vi "Nav Waveforms.vi"(10 "Log Data In":cluster{refnum<class "RDS State.lvclass">[]}[](array[cluster]), 11 "Log Header":T1) -> (2 "Log Data Out":cluster{refnum<class "RDS State.lvclass">[]}[](array[cluster]), 3 "Log Header Out":T1, 5 "Nav Data Out":waveform(dbl)[](array[waveform]))   [LabVIEW 2015, in "Log Waveform Processors.lvlib"]
uses:
  Log Waveform Processors.lvlib
  RDS State Tracker/RDS State/RDS State.lvclass
  Actors/RDS Logger Actor/RDS Logger Actor/RDS Logger Actor/Logger Header.ctl
  RDS State Tracker/RDS State/RDS State.lvclass/RDS State.ctl
  <vilib>/measure/maresamp.llb/Resample Waveform (single shot).vi
  <vilib>/Waveform/WDTFileIO.llb/Export Waveforms To Spreadsheet File (1D).vi
  <vilib>/measure/NI_MAPro.lvlib
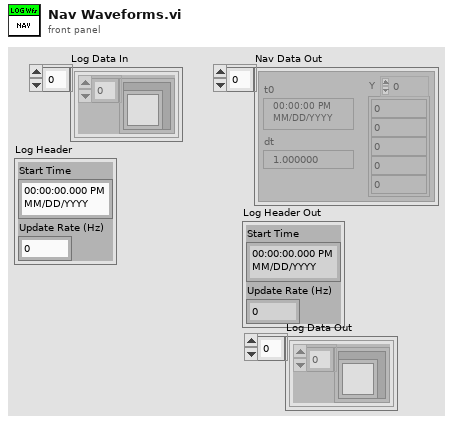
[diagram p1: front panel]
types:
  T1 = typedef "Log Waveform Processors.lvlib/Logger Header.ctl" = cluster{"Start Time":timestamp, "Update Rate (Hz)":dbl}
  T2 = typedef "RDS Libraries.lvlib/NMEA.lvlib/NMEA_GPRMC-data.ctl" = cluster{"TimeStamp":timestamp, "Validity":bool, "Latitude":dbl, "Latitude-Direction":T3, "Longitude":dbl, "Longitude-Direction":T4, "Speed in knots":sgl, "True course":sgl, "Date Stamp":timestamp, "Magnetic Variation (East/West)":sgl, "GPS Latitude":dbl, "GPS Longitude":dbl}
  T3 = typedef "RDS Libraries.lvlib/NMEA.lvlib/NMEA_LatitudeDirection.ctl" = enum16{"", "North", "South"}
  T4 = typedef "RDS Libraries.lvlib/NMEA.lvlib/NMEA_LongitudeDirection.ctl" = enum16{"", "East", "West"}
  T5 = typedef "RDS Instrument Library.lvlib/Compass Data.ctl" = cluster{"Compass Heading":sgl, "pitch Angle":sgl, "roll Angle":sgl, "Temperature":sgl, "Depth":sgl, "Magnetic Field":sgl, "Magnetic Field X":sgl, "Magnetic Field Y":sgl, "Magnetic Field Z":sgl, "Acceleration":sgl, "Acceleration X":sgl, "Acceleration Y":sgl, "Gyro":sgl, "Gyro X":sgl, "Acceleration Z":sgl, "Gyro Y":sgl, "Raw Heading":sgl}
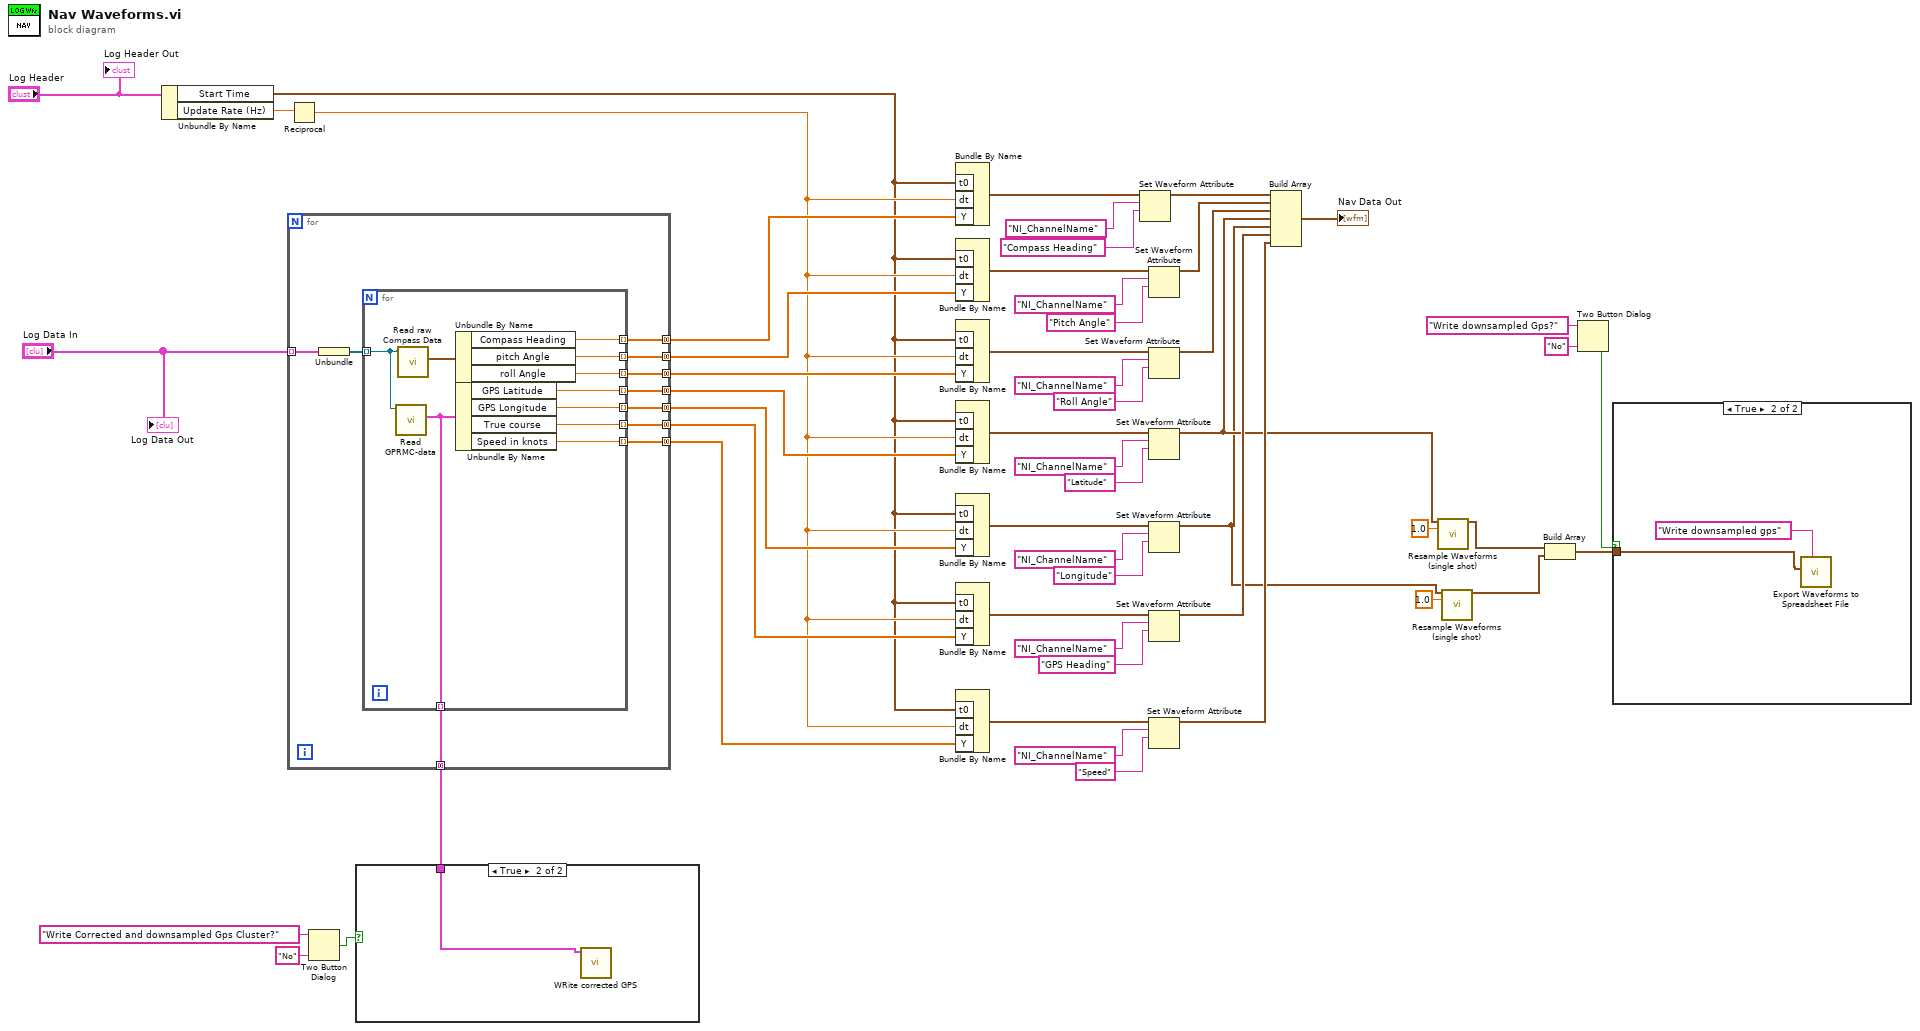
[diagram p0: block diagram]
diagram:
  n1 = Unbundle By Name("Log Header") -> ("Start Time"=w16:timestamp, "Update Rate (Hz)"=w18:dbl)
  n2 = for {
    tunnel: "Log Data In" -> [w63] mode=indexing
    tunnel: [w61] -> w25 mode=concatenating
    tunnel: [w60] -> w30 mode=concatenating
    tunnel: [w59] -> w31 mode=concatenating
    tunnel: [w58] -> w47 mode=concatenating
    tunnel: [w57] -> w48 mode=concatenating
    tunnel: [w56] -> w52 mode=concatenating
    tunnel: [w55] -> w21 mode=concatenating
    tunnel: [w54] -> w7 mode=concatenating
    n3 = Unbundle(w63) -> (w62:refnum<class "RDS State.lvclass">[])
    n4 = for {
      tunnel: w62 -> [w65] mode=indexing
      tunnel: [w73] -> w61 mode=indexing
      tunnel: [w72] -> w60 mode=indexing
      tunnel: [w71] -> w59 mode=indexing
      tunnel: [w69] -> w58 mode=indexing
      tunnel: [w68] -> w57 mode=indexing
      tunnel: [w67] -> w56 mode=indexing
      tunnel: [w66] -> w55 mode=indexing
      tunnel: [w64] -> w54 mode=indexing
      n5 = call "Read GPRMC-data.vi"("RDS State in"=w65) -> ("GPRMC-data"=w64:T2)  [unwired: 8 in, 2 out]
      n6 = call "Read raw Compass Data.vi"("RDS State in"=w65) -> ("Compass Data"=w70:T5)  [unwired: 8 in, 2 out]
      n7 = Unbundle By Name(w70) -> ("Compass Heading"=w73:sgl, "pitch Angle"=w72:sgl, "roll Angle"=w71:sgl)
      n8 = Unbundle By Name(w64) -> ("GPS Latitude"=w69:dbl, "GPS Longitude"=w68:dbl, "True course"=w67:sgl, "Speed in knots"=w66:sgl)
    }
  }
  n9 = Reciprocal(x=w18) -> (1/x=w17:dbl)
  n10 = Two Button Dialog(message="Write Corrected and downsampled Gps Cluster?", 1:"No" ("F button name (\"Cancel\")")) -> (T button?=w6:bool)  [unwired: 1 in]
  n11 = case shown="True" w6 {
    tunnel: w7 -> [_ w74]
    frame False {
    }
    frame True {
      n12 = call "WRite corrected GPS.vi"("Raw GPS Data"=w74) -> ()  [unwired: 11 in]
    }
  }
  n13 = Bundle By Name("t0"=w16, "dt"=w17, "Y"=w25) -> (w26:waveform(sgl))  [unwired: 1 in]
  n14 = Bundle By Name("t0"=w16, "dt"=w17, "Y"=w30) -> (w28:waveform(sgl))  [unwired: 1 in]
  n15 = Bundle By Name("t0"=w16, "dt"=w17, "Y"=w31) -> (w29:waveform(sgl))  [unwired: 1 in]
  n16 = Bundle By Name("t0"=w16, "dt"=w17, "Y"=w47) -> (w43:waveform(dbl))  [unwired: 1 in]
  n17 = Bundle By Name("t0"=w16, "dt"=w17, "Y"=w48) -> (w44:waveform(dbl))  [unwired: 1 in]
  n18 = Bundle By Name("t0"=w16, "dt"=w17, "Y"=w52) -> (w51:waveform(sgl))  [unwired: 1 in]
  n19 = Bundle By Name("t0"=w16, "dt"=w17, "Y"=w21) -> (w22:waveform(sgl))  [unwired: 1 in]
  n20 = Set Waveform Attribute(5:"Compass Heading" ("name"), 6:"NI_ChannelName" ("name"), 7:w26) -> (3:w32:waveform(sgl))  [unwired: 1 in, 2 out]
  n21 = Set Waveform Attribute(5:"Pitch Angle" ("name"), 6:"NI_ChannelName" ("name"), 7:w28) -> (3:w33:waveform(sgl))  [unwired: 1 in, 2 out]
  n22 = Set Waveform Attribute(5:"Roll Angle" ("name"), 6:"NI_ChannelName" ("name"), 7:w29) -> (3:w34:waveform(sgl))  [unwired: 1 in, 2 out]
  n23 = Set Waveform Attribute(5:"Latitude" ("name"), 6:"NI_ChannelName" ("name"), 7:w43) -> (3:w14:waveform(dbl))  [unwired: 1 in, 2 out]
  n24 = Set Waveform Attribute(5:"Longitude" ("name"), 6:"NI_ChannelName" ("name"), 7:w44) -> (3:w11:waveform(dbl))  [unwired: 1 in, 2 out]
  n25 = Set Waveform Attribute(5:"GPS Heading" ("name"), 6:"NI_ChannelName" ("name"), 7:w51) -> (3:w53:waveform(sgl))  [unwired: 1 in, 2 out]
  n26 = Set Waveform Attribute(5:"Speed" ("name"), 6:"NI_ChannelName" ("name"), 7:w22) -> (3:w15:waveform(sgl))  [unwired: 1 in, 2 out]
  n27 = Build Array(w32, w33, w34, w14, w11, w53, w15) -> (→"Nav Data Out":waveform(dbl)[])
  n28 = call-poly <vilib>:"Resample Waveforms (single shot).vi"("waveform in"=w14, "dt"=1.0) -> ("resampled waveform out"=w10:waveform(dbl))  [unwired: 10 in, 3 out]
  n29 = call-poly <vilib>:"Resample Waveforms (single shot).vi"("waveform in"=w11, "dt"=1.0) -> ("resampled waveform out"=w9:waveform(dbl))  [unwired: 10 in, 3 out]
  n30 = Build Array(w10, w9) -> (w8:waveform(dbl)[])
  n31 = Two Button Dialog(message="Write downsampled Gps?", 1:"No" ("F button name (\"Cancel\")")) -> (T button?=w3:bool)  [unwired: 1 in]
  n32 = case shown="True" w3 {
    tunnel: w8 -> [_ w76]
    frame False {
    }
    frame True {
      n33 = call-poly <vilib>:"Export Waveforms to Spreadsheet File.vi"("prompt"="Write downsampled gps", "waveforms"=w76) -> ()  [unwired: 8 in, 2 out]
    }
  }
  "Log Header Out" <- "Log Header"
  "Log Data Out" <- "Log Data In"
